vi "Read Path DB.vi"(8 "error in (no error)":errorcluster, 11 "DB in":refnum<class "DB.lvclass">) -> (0 "error out":errorcluster, 2 "Path DB":path, 3 "DB out":refnum<class "DB.lvclass">)   [LabVIEW 2015, in "DB.lvclass"]
uses:
  DB.lvclass
  DB.lvclass/DB.ctl
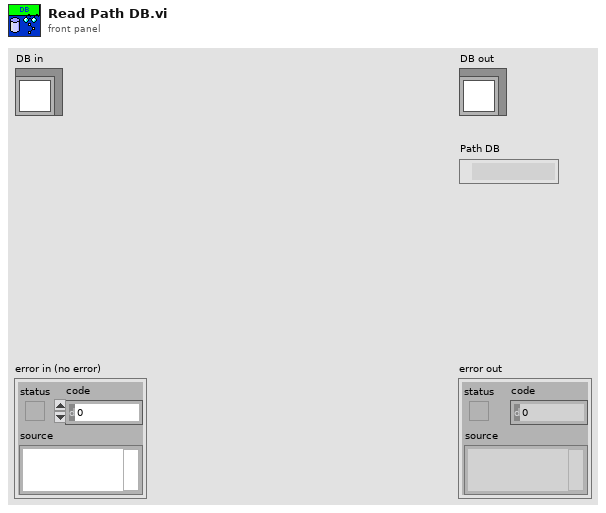
[diagram p1: front panel]
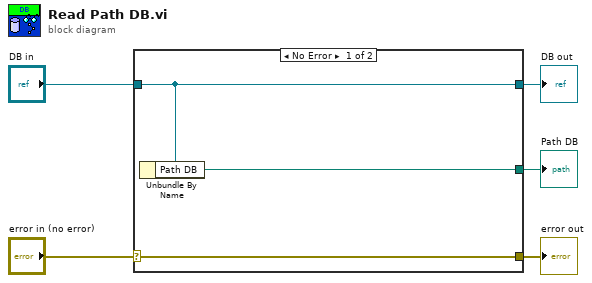
[diagram p0: block diagram]
diagram:
  n1 = case shown="No Error" "error in (no error)" {
    selector: "error in (no error)" -> [w8 w9]
    tunnel: [w8 w9] -> w4
    tunnel: [w7 w10] -> w2
    tunnel: "DB in" -> [w7 w10]
    tunnel: [w6 _] -> w1
    frame No Error {
      n2 = Unbundle By Name(w7) -> ("Path DB"=w6:path)
    }
    frame Error {
    }
  }
  "error out" <- w4
  "DB out" <- w2
  "Path DB" <- w1
